vi "AssetMgrGetAssetNodeCountForDefinitionResponse_Name.vi"() -> (1 "MessageName":string)   [LabVIEW 2017]
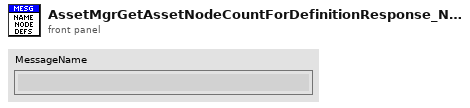
[diagram p1: front panel]
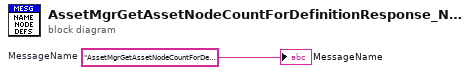
[diagram p0: block diagram]
diagram:
  w1 = "AssetMgrGetAssetNodeCountForDefinitionResponse"  # MessageName
  "MessageName" <- w1
